vi "System Explorer - Copy Templates for System Explorer.vi"(7 "CD Name":string, 8 "error in (no error)":errorcluster, 11 "System Explorer folder":path) -> (0 "error out":errorcluster)   [LabVIEW 2015, in "NIVS_Consolidated_CDW_MetaDataObj.lvclass"]
doc: "Copy the templates for the System Explorer library into the System Explorer folder and disconnect the templates from the owning library."
uses:
  NIVS_Consolidated_CDW_MetaDataObj.lvclass
  CD System Explorer lvlib.ctl
  Common.ctl
  CD Shared lvlib.ctl
  CD System Explorer lvlib.vi
  Common.vi
  CD Shared lvlib.vi
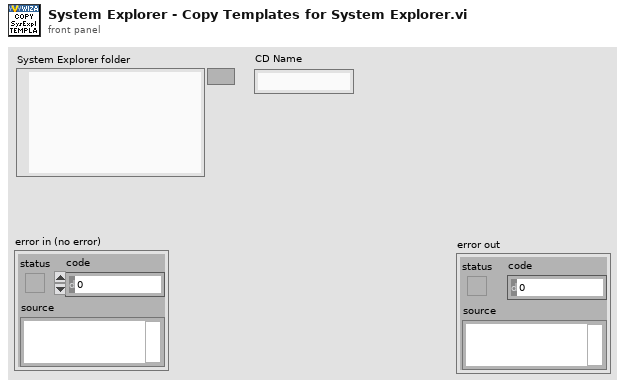
[diagram p1: front panel]
types:
  T1 = typedef "NIVS_Consolidated_CDW_MetaDataObj.lvclass/CD System Explorer lvlib.ctl" = enum16{"LibraryFileName", "LibraryFolderName", "System Explorer.FolderName", "System Explorer.Dynamically Called.FolderName", "System Explorer.Dynamically Called.Extra Pages.FolderName", "System Explorer.Dynamically Called.Extra Pages.TemplatePathAndName", "System Explorer.Dynamically Called.Main Page.VIName", "System Explorer.Dynamically Called.Main Page.TemplatePathAndName", "System Explorer.Dynamically Called.Initialization VI.VIName", "System Explorer.Dynamically Called.Initialization VI.TemplatePathAndName", "System Explorer.SubVI.FolderName", "System Explorer.Types.FolderName", "System Explorer.ActionVIOnCompile.VIName", "System Explorer.ExportConfigRTM.VIName", "System Explorer.LoadHelpFile.VIName"}
  T2 = typedef "NIVS_Consolidated_CDW_MetaDataObj.lvclass/CD Shared lvlib.ctl" = enum16{"LibraryFileName", "LibraryFolderName", "ConstantsVI.VIPathAndName", "Shared.FolderName", "Shared.Types.FolderName", "Shared.Constants.VIName", "Shared.Constants.VITemplateName", "Shared.Constants.VITemplatePathAndName", "Shared.CompiledSettings.RelativePath", "Shared.Constants.RelativePath", "Shared.CompiledSettings.Name", "Shared.CompiledSettings.Name.NoExtension", "Shared.CompiledSettings.ClusterName"}
  T3 = typedef "NIVS_Consolidated_CDW_MetaDataObj.lvclass/Common.ctl" = enum16{"ProjectName", "TemplatesFolderName", "ProjectTemplatePathAndName", "TimingAndSyncFolderName", "CustomDeviceFolderName", "PathToTemplates"}
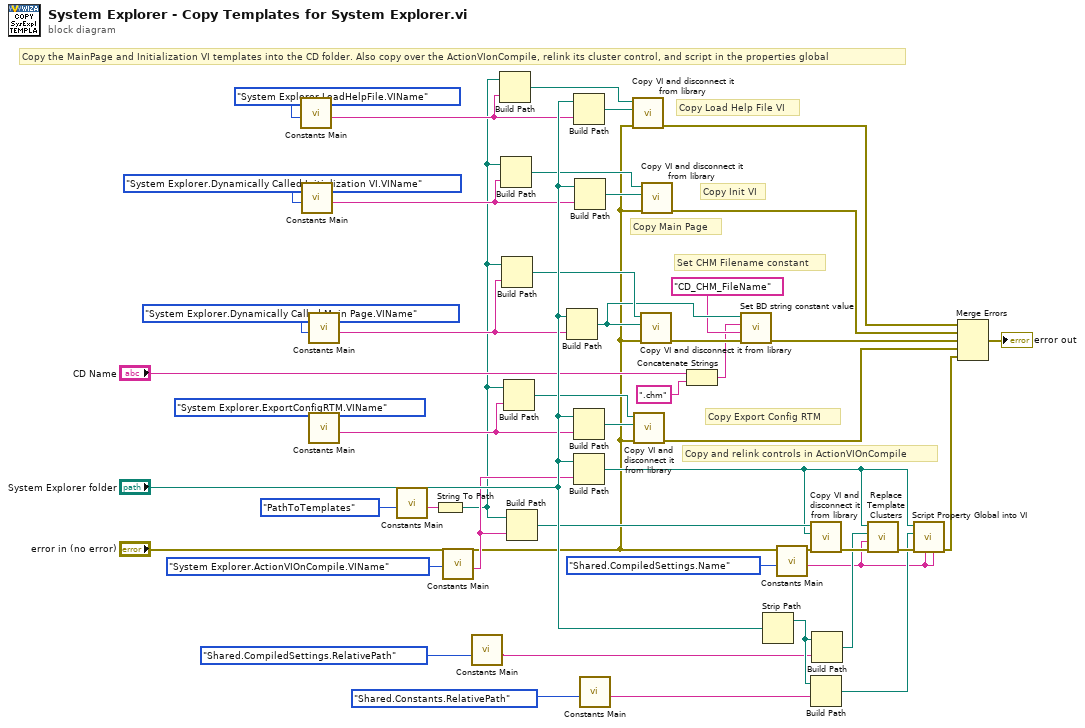
[diagram p0: block diagram]
diagram:
  # "Copy Load Help File VI"
  # "Copy the MainPage and Initialization VI templates into the CD folder. Also copy over the ActionVIonCompile, relink its cluster control, and script in the properties global"
  # "Set CHM Filename constant"
  # "Copy Export Config RTM"
  # "Copy and relink controls in ActionVIOnCompile"
  # "Copy Main Page"
  # "Copy Init VI"
  n1 = call-poly "Constants Main.vi"("Action"=CD_System_Explorer_lvlib."System Explorer.LoadHelpFile.VIName") -> ("Output"=w7:string)  [unwired: 10 in]
  n2 = call-poly "Constants Main.vi"("Action"=CD_System_Explorer_lvlib."System Explorer.Dynamically Called.Initialization VI.VIName") -> ("Output"=w35:string)  [unwired: 10 in]
  n3 = call-poly "Constants Main.vi"("Action"=CD_System_Explorer_lvlib."System Explorer.Dynamically Called.Main Page.VIName") -> ("Output"=w34:string)  [unwired: 10 in]
  n4 = call-poly "Constants Main.vi"("Action"=CD_System_Explorer_lvlib."System Explorer.ExportConfigRTM.VIName") -> ("Output"=w17:string)  [unwired: 10 in]
  n5 = call-poly "Constants Main.vi"("Action"=Common."PathToTemplates") -> ("Output"=w40:string)  [unwired: 10 in]
  n6 = String To Path(string=w40) -> (path=w3:path)
  n7 = call-poly "Constants Main.vi"("Action"=CD_System_Explorer_lvlib."System Explorer.ActionVIOnCompile.VIName") -> ("Output"=w27:string)  [unwired: 10 in]
  n8 = call-poly "Constants Main.vi"("Action"=CD_Shared_lvlib."Shared.CompiledSettings.RelativePath") -> ("Output"=w25:string)  [unwired: 10 in]
  n9 = Build Path(base path=w3, name or relative path=w7) -> (appended path=w6:path)
  n10 = Build Path(base path=w3, name or relative path=w35) -> (appended path=w36:path)
  n11 = Build Path(base path=w3, name or relative path=w34) -> (appended path=w37:path)
  n12 = Build Path(base path=w3, name or relative path=w17) -> (appended path=w20:path)
  n13 = Build Path(base path=w3, name or relative path=w27) -> (appended path=w39:path)
  n14 = Build Path(base path="System Explorer folder", name or relative path=w34) -> (appended path=w13:path)
  n15 = Build Path(base path="System Explorer folder", name or relative path=w7) -> (appended path=w5:path)
  n16 = Build Path(base path="System Explorer folder", name or relative path=w17) -> (appended path=w19:path)
  n17 = Build Path(base path="System Explorer folder", name or relative path=w27) -> (appended path=w32:path)
  n18 = Build Path(base path="System Explorer folder", name or relative path=w35) -> (appended path=w43:path)
  n19 = call-poly "Constants Main.vi"("Action"=CD_Shared_lvlib."Shared.Constants.RelativePath") -> ("Output"=w23:string)  [unwired: 10 in]
  n20 = call "Copy VI and disconnect it from library.vi"("error in (no error)"="error in (no error)", "VI Target Path"=w5, "VI Source Path"=w6) -> ("error out"=w2:errorcluster)  [unwired: 8 in]
  n21 = call "Copy VI and disconnect it from library.vi"("error in (no error)"="error in (no error)", "VI Target Path"=w19, "VI Source Path"=w20) -> ("error out"=w15:errorcluster)  [unwired: 8 in]
  n22 = call "Copy VI and disconnect it from library.vi"("error in (no error)"="error in (no error)", "VI Target Path"=w13, "VI Source Path"=w37) -> ("error out"=w14:errorcluster)  [unwired: 8 in]
  n23 = call "Copy VI and disconnect it from library.vi"("error in (no error)"="error in (no error)", "VI Target Path"=w43, "VI Source Path"=w36) -> ("error out"=w42:errorcluster)  [unwired: 8 in]
  n24 = Concatenate Strings("CD Name", ".chm" ("string")) -> (w9:string)
  n25 = call "Set BD string constant value.vi"("error in (no error)"=w14, "Name of string constant"="CD_CHM_FileName", "New String Value"=w9, "Path to VI"=w13) -> ("error out"=w11:errorcluster)  [unwired: 7 in]
  n26 = Strip Path(path="System Explorer folder") -> (stripped path=w30:path)  [unwired: 1 out]
  n27 = call-poly "Constants Main.vi"("Action"=CD_Shared_lvlib."Shared.CompiledSettings.Name") -> ("Output"=w22:string)  [unwired: 10 in]
  n28 = call "Copy VI and disconnect it from library.vi"("error in (no error)"="error in (no error)", "VI Target Path"=w32, "VI Source Path"=w39) -> ("error out"=w38:errorcluster)  [unwired: 8 in]
  n29 = Build Path(base path=w30, name or relative path=w23) -> (appended path=w29:path)
  n30 = Build Path(base path=w30, name or relative path=w25) -> (appended path=w31:path)
  n31 = call "Replace Template Clusters.vi"("error in (no error)"=w38, "Control Name"=w22, "Path to Cluster to Replace"=w31, "Path to VI"=w32) -> ("error out"=w33:errorcluster)  [unwired: 7 in]
  n32 = call "Script Property Global into VI.vi"("GlobalControlName"=w22, "StringConstantToReplace"=w22, "error in (no error)"=w33, "Path to Global"=w29, "Path to VI"=w32) -> ("error out"=w16:errorcluster)  [unwired: 6 in]
  n33 = Merge Errors(w2, w42, w11, w15, w16) -> (→"error out":errorcluster)
